vi "Eth Status Write Start.vi"(7 "Status Reference":T1, 8 "error in (no error)":errorcluster, 9 "Start":bool, 11 "N":i32) -> (0 "error out":errorcluster)   [LabVIEW 2021, in "Eth Status.lvlib"]
uses:
  Eth Status.lvlib
  Ctl/Status.ctl
  MB_TCP2/MB_TCP_State.ctl
  MB_TCP2/MB_TCP.lvclass
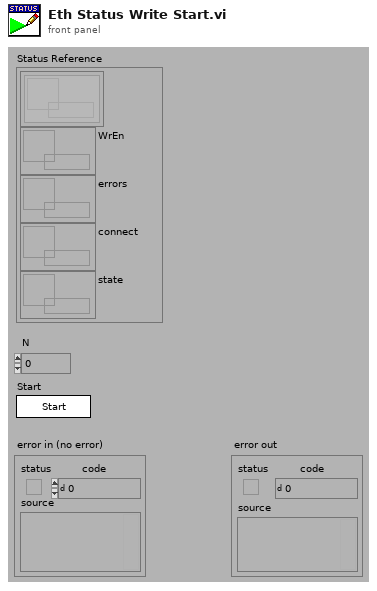
[diagram p1: front panel]
types:
  T1 = typedef "Eth Status.lvlib/Status.ctl" = cluster{"Set_states":refnum<queue>[], "WrEn":refnum<data-value>, "errors":refnum<data-value>, "connect":refnum<data-value>, "state":refnum<data-value>}
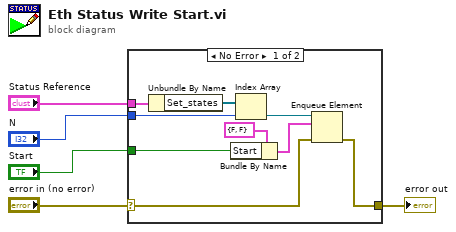
[diagram p0: block diagram]
diagram:
  n1 = case shown="No Error" "error in (no error)" {
    selector: "error in (no error)" -> [w14 w15]
    tunnel: [w12 w15] -> w2
    tunnel: "Status Reference" -> [w11 _]
    tunnel: "Start" -> [w13 _]
    tunnel: "N" -> [w7 _]
    frame No Error {
      n2 = Unbundle By Name(w11) -> ("Set_states"=w8:refnum<queue>[])
      n3 = Bundle By Name(cluster=cluster{"Start":bool, "Stop":bool} {"Start"=FALSE, "Stop"=FALSE} ("element"), "Start"=w13) -> (w9:cluster{"Start":bool, "Stop":bool})
      n4 = Index Array(array=w8, index=w7) -> (element=w6:refnum<queue>)
      n5 = Enqueue Element(queue=w6, element=w9, error in (no error)=w14) -> (error out=w12:errorcluster)  [unwired: 1 in, 2 out]
    }
    frame Error {
    }
  }
  "error out" <- w2
